vi "Enable disable buttons.vi"(7 "enable?":bool=TRUE, 8 "error in (no error)":errorcluster, 11 "references":refnum<vi>[](array[refnum])) -> (0 "error out":errorcluster)   [LabVIEW 2012, in "ServiceManager.lvclass"]
doc: "Enables the control when the boolean 'Enable?' is TRUE and disables and grays out the control when the value is FALSE."
uses:
  ServiceManager.lvclass
  <vilib>/Distrio/Murmex/Murmex/Murmex.lvclass
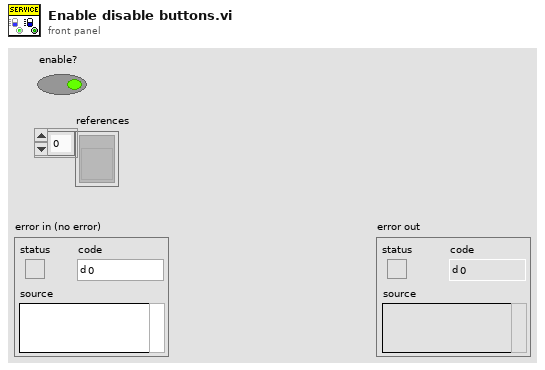
[diagram p1: front panel]
types:
  T1 = enum8{"Enabled", "Disabled", "Disabled and Grayed Out"}
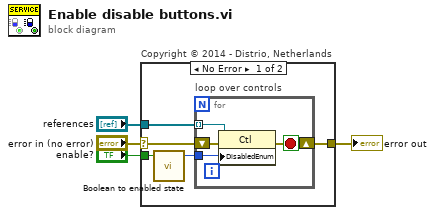
[diagram p0: block diagram]
diagram:
  n1 = case "Copyright © 2014 - Distrio, Netherlands" shown="No Error" "error in (no error)" {
    selector: "error in (no error)" -> [w5 w14]
    tunnel: "enable?" -> [w9 _]
    tunnel: "references" -> [w8 _]
    tunnel: [w6 w14] -> w2
    frame No Error {
      n2 = call <vilib>:"Boolean to enabled state.vi"("boolean in"=w9) -> ("enabled status out"=w7:T1)  [unwired: 4 in]
      n3 = for "loop over controls" {
        tunnel: w8 -> [w13] mode=indexing
        tunnel: w7 -> [w11]
        shift-right: [w10] -> w6
        shift-left: w5 -> [w12]
        stop <- w10 stop-if-true
        n4 = property class="Ctl"(reference=w13, error in=w12, "DisabledEnum"=w11) -> (error out=w10:errorcluster)  [unwired: 1 out]
      }
    }
    frame Error {
    }
  }
  "error out" <- w2
